vi "image_copy.vi"(10 "buffer name":string, 11 "image in":T1) -> (3 "imgae out":T1)   [LabVIEW 2017]
uses:
  <vilib>/vision/Image Controls.llb/IMAQ Image.ctl
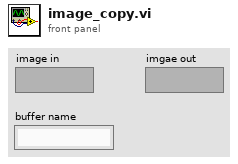
[diagram p1: front panel]
types:
  T1 = typedef "IMAQ Image.ctl" = refnum<image>
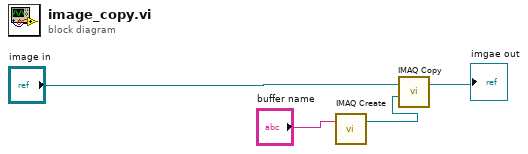
[diagram p0: block diagram]
diagram:
  n1 = call "IMAQ Create"("Image Name"="buffer name") -> ("New Image"=w1:T1)  [unwired: 4 in, 1 out]
  n2 = call "IMAQ Copy"("Image Dst"=w1, "Image Src"="image in") -> ("Image Dst Out"=→"imgae out":T1)  [unwired: 4 in, 1 out]
